vi "Chroma 1905x Series System Lock Owner Query.vi"(8 "error in (no error)":errorcluster, 11 "VISA resource name":refnum<visa-resource-name>) -> (0 "error out":errorcluster, 3 "VISA resource name out":refnum<visa-resource-name>)   [LabVIEW 2025]
panel:
  out "Owner":string
  # "Lock Owner query"
  # "1 means RMT (Remote)"
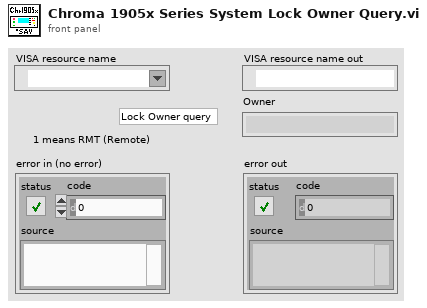
[diagram p1: front panel]
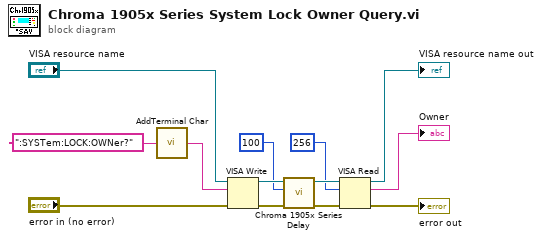
[diagram p0: block diagram]
diagram:
  n1 = call "AddTerminal Char.vi"("Cmd string"=":SYSTem:LOCK:OWNer?") -> ("Concatenated String"=w5:string)  [unwired: 4 in]
  n2 = VISA Write(VISA resource name="VISA resource name", write buffer=w5, error in (no error)="error in (no error)") -> (VISA resource name out=w10:refnum<visa-resource-name>, error out=w12:errorcluster)  [unwired: 1 out]
  n3 = call "Chroma 1905x Series Delay.vi"("error in (no error)"=w12, "Time Delay [ms]"=u32 100 ("Time Delay ms"), "VISA resource name"=w10) -> ("error out"=w11:errorcluster, "VISA resource name 2"=w9:refnum<visa-resource-name>)  [unwired: 7 in]
  n4 = VISA Read(VISA resource name=w9, byte count=u32 256, error in (no error)=w11) -> (VISA resource name out=→"VISA resource name out":refnum<visa-resource-name>, read buffer=→"Owner":string, error out=→"error out":errorcluster)  [unwired: 1 out]
